vi "Error 0 (SubVI).vi"(0 "array type (2D Dbl)":i32[][](array[numeric])) -> (7 "Numeric":i32, 8 "Numeric 6":i32, 11 "Numeric 3":i32, 14 "Numeric 5":i32, 15 "Numeric 2":i32, 16 "result":bool, 18 "Numeric 4":i32)   [LabVIEW 2015]
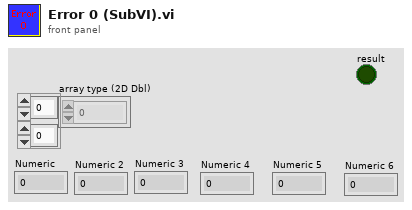
[diagram p1: front panel]
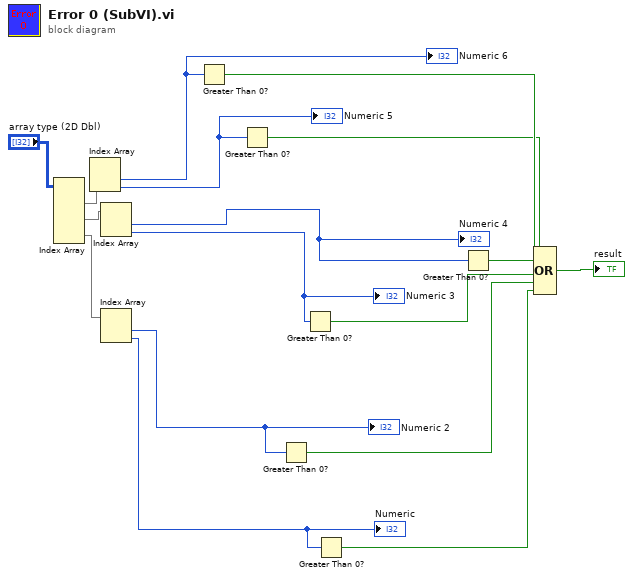
[diagram p0: block diagram]
diagram:
  n1 = Index Array(array="array type (2D Dbl)") -> (element #1=w13:i32[], element #2=w14:i32[], element #3=w15:i32[])  [unwired: 6 in]
  n2 = Index Array(array=w13) -> (element #1=w16:i32, element #2=w17:i32)  [unwired: 2 in]
  "Numeric 5" <- w17
  "Numeric 6" <- w16
  n3 = Index Array(array=w14) -> (element #1=w9:i32, element #2=w8:i32)  [unwired: 2 in]
  "Numeric 3" <- w8
  "Numeric 4" <- w9
  n4 = Index Array(array=w15) -> (element #1=w10:i32, element #2=w11:i32)  [unwired: 2 in]
  "Numeric" <- w11
  "Numeric 2" <- w10
  n5 = Greater Than 0?(x=w16) -> (x > 0?=w7:bool)
  n6 = Greater Than 0?(x=w17) -> (x > 0?=w6:bool)
  n7 = Greater Than 0?(x=w10) -> (x > 0?=w3:bool)
  n8 = Greater Than 0?(x=w8) -> (x > 0?=w4:bool)
  n9 = Greater Than 0?(x=w11) -> (x > 0?=w2:bool)
  n10 = Greater Than 0?(x=w9) -> (x > 0?=w5:bool)
  n11 = Compound Arithmetic op=OR(w7, w6, w5, w4, w3, w2) -> (→"result":bool)
